vi "ROI group-Update single group info.vi"(8 "error in (no error)":errorcluster, 9 "Index of renamed group":i32, 11 "POI group info cluster":T1 {"Group region specifier cluster"."Contours"."Type" items=["No Selection", "Point", "Line", "Rectangle", "Oval", "Polygon", "Freehand Region", "Annulus", "Unused2", "Unused3", "Broken Line", "Freehand Line", "Rotated Rectangle"]}) -> (0 "error out":errorcluster, 2 "Updated \"All groups\" setup":T1[](array[typedef]) {"Group region specifier cluster"."Contours"."Type" items=["No Selection", "Point", "Line", "Rectangle", "Oval", "Polygon", "Freehand Region", "Annulus", "Unused2", "Unused3", "Broken Line", "Freehand Line", "Rotated Rectangle"]})   [LabVIEW 2013]
uses:
  ROI Selection Interface/ROI group info cluster.ctl
  Typedefs/Get-Set-Clear Control.ctl
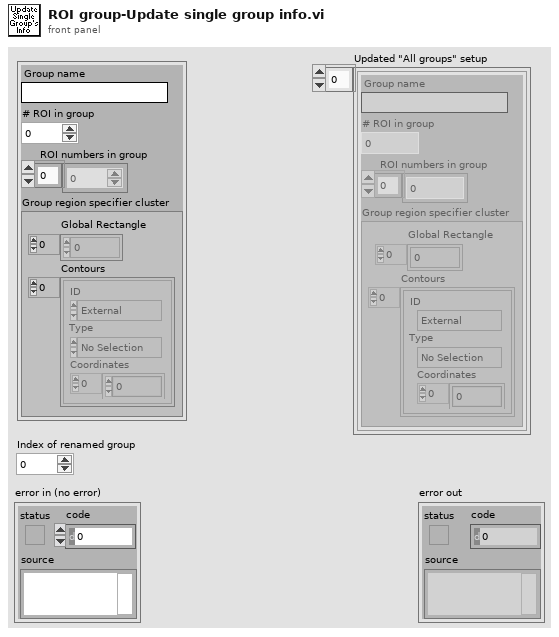
[diagram p1: front panel]
types:
  T1 = typedef "ROI group info cluster.ctl" = cluster{"Group name":string, "# ROI in group":i32, "ROI numbers in group":i32[], "Group region specifier cluster":T2}
  T2 = typedef "ROI Descriptor" = cluster{"Global Rectangle":i32[], "Contours":cluster{"ID":enum32{"External", "Internal"}, "Type":u32, "Coordinates":i32[]}[]}
  T3 = typedef "Get-Set-Clear Control.ctl" = enum16{"Get", "Set", "Clear"}
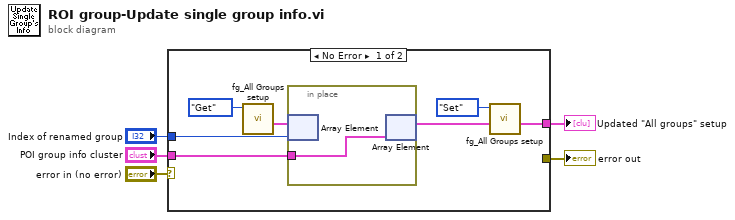
[diagram p0: block diagram]
diagram:
  n1 = case shown="No Error" "error in (no error)" {
    selector: "error in (no error)" -> [_ w14]
    tunnel: "POI group info cluster" -> [w7 _]
    tunnel: [w10 _] -> w5
    tunnel: [_ w14] -> w3
    tunnel: "Index of renamed group" -> [w8 _]
    frame No Error {
      n2 = call "fg_All Groups setup.vi"("Function"=Get-Set-Clear_Control."Get") -> ("Groups setup out"=w9:T1[])  [unwired: 9 in, 1 out]
      n3 = in-place {
        in-place-border: w7 -> [w13]
        n4 = in-place-array #1(w9, w8) -> ()  [unwired: 1 out]
        n5 = in-place-array #1(w13) -> (w6:T1[])  [unwired: 1 out]
      }
      n6 = call "fg_All Groups setup.vi"("Groups setup in"=w6, "Function"=Get-Set-Clear_Control."Set") -> ("Groups setup out"=w10:T1[])  [unwired: 8 in, 1 out]
    }
    frame Error {
    }
  }
  "Updated \"All groups\" setup" <- w5
  "error out" <- w3
